vi "Wait till Interval.vi"(8 "error in (no error)":errorcluster, 11 "Function in":refnum<class "Function.lvclass">) -> (0 "error out":errorcluster, 3 "Function out":refnum<class "Function.lvclass">)   [LabVIEW 2016, in "Function Actor.lvlib" / "Function.lvclass"]
uses:
  <userlib>/Common Components/Function Actor/Function.lvclass
  <userlib>/Common Components/Function Actor/Function.lvclass/Function.ctl
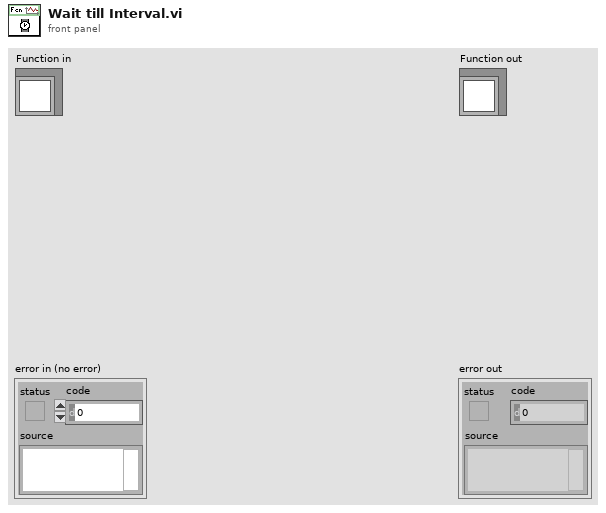
[diagram p1: front panel]
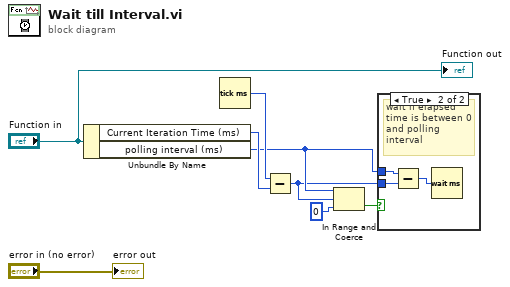
[diagram p0: block diagram]
diagram:
  n1 = Unbundle By Name("Function in") -> ("Current Iteration Time (ms)"=w5:u32, "polling interval (ms)"=w2:u32)
  n2 = Tick Count (ms)() -> (millisecond timer value=w6:u32)
  n3 = Subtract(x=w6, y=w5) -> (x-y=w1:u32)
  n4 = In Range and Coerce(upper limit=w2, x=w1, lower limit=u32 0) -> (In Range?=w3:bool)  [unwired: 1 out]
  n5 = case shown="True" w3 {
    tunnel: w2 -> [_ w11]
    tunnel: w1 -> [_ w10]
    frame False {
    }
    frame True {
      # "wait if elapsed time is between 0 and polling interval"
      n6 = Subtract(x=w11, y=w10) -> (x-y=w9:u32)
      n7 = Wait (ms)(milliseconds to wait=w9) -> ()  [unwired: 1 out]
    }
  }
  "error out" <- "error in (no error)"
  "Function out" <- "Function in"
